vi "Core Action.vi"(8 "error in (no error)":errorcluster, 10 "SECS-II Class In":refnum<class "SECS-II Class.lvclass">, 11 "33-RPTID Setup in":refnum<class "33-RPTID Setup.lvclass">) -> (0 "error out":errorcluster, 2 "SECS-II Class Out":refnum<class "SECS-II Class.lvclass">, 3 "33-RPTID Setup out":refnum<class "33-RPTID Setup.lvclass">)   [LabVIEW 2020, in "SECS Scenarios.lvlib" / "33-RPTID Setup.lvclass"]
uses:
  33-RPTID Setup.lvclass
  D:/Dropbox/SECS/SECS_GEM v1.1.0/Com/SECS Scenarios/Scenarios Class/Scenarios Class.lvclass
  SECS Communication/SECS-II Class/SECS-II Class.lvclass
  SECS Communication/S2 Message Class/S2 Message Class.lvclass
  D:/Dropbox/SECS/SECS_GEM v1.1.0/Com/SECS Communication/SECS-II Class/SECS-II Class.lvclass
  Scenarios Class/Reply State.ctl
  Scenarios Class/Scenarios Class.lvclass/Scenarios Class.ctl
  Scenarios Class/Write Reply State.vi
  Scenarios Class/Read HSMS Class.vi
  SECS Communication/HSMS Class/HSMS Class.lvclass
  Scenarios Class/Scenarios Class.lvclass
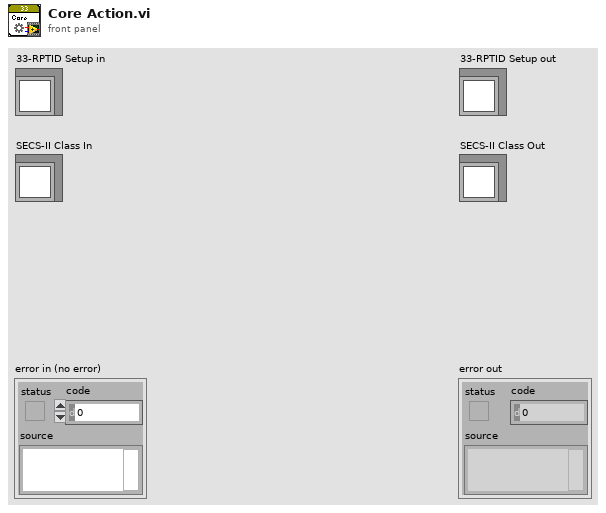
[diagram p1: front panel]
types:
  T1 = typedef "SECS Communication.lvlib/S2 Message Class.lvclass/S2F33.ctl" = cluster{"DATAID":u32, "RPTID Data":cluster{"RPTID":u32, "VID":u32[]}[]}
  T2 = typedef "SECS Scenarios.lvlib/Scenarios Class.lvclass/Reply State.ctl" = enum16{"OK", "Illegal Data", "Unknown Stream", "Unknown Function", "Off-Line", "T3 Timeout", "Inner-Timeout"}
  T3 = typedef "SECS Communication.lvlib/S2 Message Class.lvclass/S2F34.ctl" = enum16{"ok", "out of space", "invalid format", "1 or more RPTID already defined", "1 or more invalid VID"}
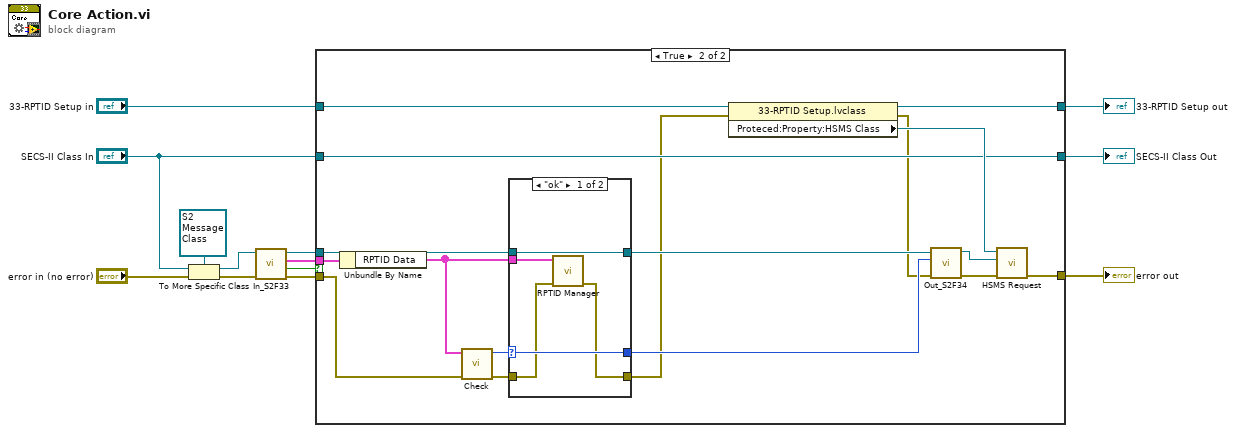
[diagram p0: block diagram]
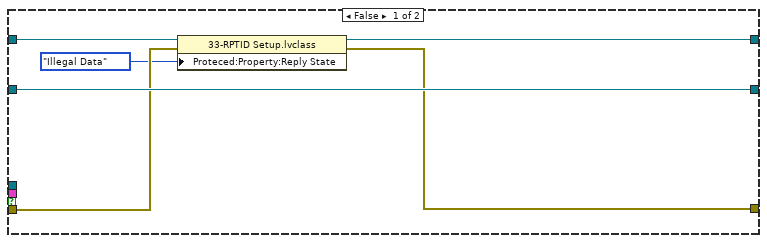
[diagram p2: hidden frame]
diagram:
  n1 = To More Specific Class(target class=refnum<class "S2 Message Class.lvclass"> refnum ("S2 Message Class in"), reference="SECS-II Class In", error in="error in (no error)") -> (specific class reference=w11:refnum<class "S2 Message Class.lvclass">, error out=w12:errorcluster)
  n2 = call "In_S2F33.vi"("error in (no error)"=w12, "S2 Message Class in"=w11) -> ("error out"=w9:errorcluster, "OK?"=w10:bool, "S2F33"=w8:T1, "S2 Message Class out"=w7:refnum<class "S2 Message Class.lvclass">)  [unwired: 6 in]
  n3 = case shown="True" w10 {
    tunnel: w9 -> [w17 w29]
    tunnel: w8 -> [_ w21]
    tunnel: w7 -> [_ w26]
    tunnel: "33-RPTID Setup in" -> [w18 w36]
    tunnel: "SECS-II Class In" -> [w19 w33]
    tunnel: [w15 w34] -> w1
    tunnel: [w19 w33] -> w2
    tunnel: [w14 w32] -> w3
    frame False {
      n4 = property class="33-RPTID Setup.lvclass"(reference=w18, error in=w17, "Proteced:Property:Reply State"=Reply_State."Illegal Data" ("Reply State")) -> (reference out=w15:refnum<class "33-RPTID Setup.lvclass">, error out=w14:errorcluster)
    }
    frame True {
      n5 = Unbundle By Name(w21) -> ("RPTID Data"=w20:cluster{"RPTID":u32, "VID":u32[]}[])
      n6 = call "Check.vi"("error in (no error)"=w29, "RPTID Data"=w20) -> ("error out"=w28:errorcluster, "S2F34"=w27:T3)  [unwired: 8 in]
      n7 = case shown="\"ok\"" w27 {
        selector: w27 -> [w40 w43]
        tunnel: w28 -> [w38 w44]
        tunnel: w26 -> [w41 w42]
        tunnel: [w37 w44] -> w23
        tunnel: [w40 w43] -> w25
        tunnel: [w41 w42] -> w24
        tunnel: w20 -> [w39 _]
        frame "ok" {
          n8 = call "RPTID Manager.vi"("error in (no error)"=w38, "RPTID Data"=w39) -> ("error out"=w37:errorcluster)  [unwired: 9 in]
        }
        frame Default {
        }
      }
      n9 = property class="33-RPTID Setup.lvclass"(reference=w36, error in=w23) -> (reference out=w34:refnum<class "33-RPTID Setup.lvclass">, error out=w22:errorcluster, "Proteced:Property:HSMS Class"=w35:refnum<class "HSMS Class.lvclass">)
      n10 = call "Out_S2F34.vi"("error in (no error)"=w22, "S2F34"=w25, "S2 Message Class in"=w24) -> ("error out"=w30:errorcluster, "S2 Message Class out"=w31:refnum<class "S2 Message Class.lvclass">)  [unwired: 7 in]
      n11 = call "HSMS Request.vi"("error in (no error)"=w30, "SECS-II Class In"=w31, "HSMS Class in"=w35) -> ("error out"=w32:errorcluster)  [unwired: 7 in, 1 out]
    }
  }
  "error out" <- w3
  "33-RPTID Setup out" <- w1
  "SECS-II Class Out" <- w2
